vi "ABR3-Threshold To String.vi"(1 "Threshold":dbl) -> (0 "String":string)   [LabVIEW 2020]
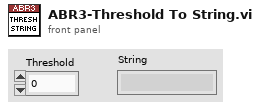
[diagram p1: front panel]
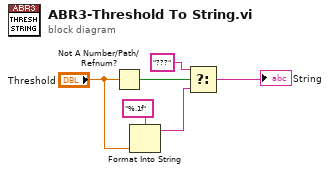
[diagram p0: block diagram]
diagram:
  n1 = Not A Number/Path/Refnum?(number/path/refnum="Threshold") -> (NaN/Path/Refnum?=w6:bool)
  n2 = Format Into String(format string="%.1f", "Threshold") -> (resulting string=w3:string)  [unwired: 2 in, 1 out]
  n3 = Select(t="???", s=w6, f=w3) -> (s? t:f=→"String":string)
